vi "Pre Launch Init.vi"(11 "Image Acquisition in":refnum<class "Image Acquisition.lvclass">) -> (0 "error out":errorcluster, 3 "Image Acquisition out":refnum<class "Image Acquisition.lvclass">)   [LabVIEW 2019, in "Image Acquisition.lvlib" / "Image Acquisition.lvclass"]
doc: "(<B>Filename</B>: Actor Framework.lvlib:Actor.lvclass:Pre Launch Init.vi)\n\nDefines behavior that occurs after the Launch Nested Actor method is invoked but before the actor's Actor Core method begins running.\n\nBy default, this method does nothing. A descendant class may override it to define behavior."
uses:
  Image Acquisition.lvclass
  <vilib>/vision/Image Controls.llb/IMAQ Image.ctl
  TypeDefs/Acquired Image Info.ctl
  <vilib>/userdefined/High Color/IMAQdx.ctl
  <vilib>/vision/driver/IMAQdx.llb/IMAQdx Acquisition Mode.ctl
  <vilib>/vision/driver/IMAQdx.llb/IMAQdx Buffer Number Mode.ctl
  TypeDefs/Image Acquisition Parameters.ctl
  TypeDefs/Initialize Data IA.ctl
  <vilib>/ActorFramework/Actor/Actor.lvclass
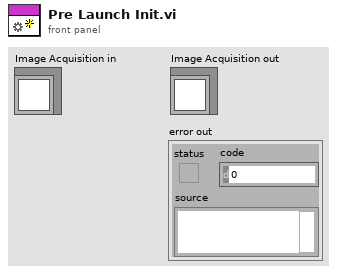
[diagram p1: front panel]
types:
  T1 = typedef "Image Acquisition.lvlib/Image Acquisition.lvclass/Initialize Data IA.ctl" = cluster{"Core":cluster{"Current VI Reference":refnum<vi>, "Close Panel on Exit?":bool}, "IA JSON File Path":path, "Buffer Number":u64, "Missed Frame Count":i32, "Timeout":i32, "Image_Counter_CA":u64, "Imaqdx Session In":T2, "filenames":string[], "File path to read images":path, "Sequence":string, "IMAQ ring Buffer":T3[], "Buffer count":i32, "AOI":i32[], "Offline Images Ring Buffer":T3[], "ReceiverSequence":cluster{"ReceiverID":i32, "Index":i32}[], "Number Of Buffers":i32, "IMAQ Offline Image Buffer":T3[], "IMAQ Run image Buffer ":T3[], "Camera parameters":T4, "CurrentPartParameters":cluster{"Name":string, "ReceiverSequence":cluster{"ReceiverID":dbl, "Index":dbl}[], "AOI":i32[], "filePath":string}, "Exposure Time":u32, "File path @ Run":path, "State Ack":cluster{"State":string, "Status":string}}
  T2 = typedef "IMAQdx.ctl" = refnum<k21>
  T3 = typedef "IMAQ Image.ctl" = refnum<image>
  T4 = typedef "Image Acquisition.lvlib/Image Acquisition.lvclass/Image Acquisition Parameters.ctl" = cluster{"Camera parameters":cluster{"Id":i32, "Type":string, "Model":string, "InterfaceType":string, "SerialNumber":string, "Timeout":i32, "NumberOfBuffers":i32, "AcquisitionTimeout":i32, "ImageName":string, "ColorCameraParam":cluster{"PixelFormat":string, "GammaEnable":bool, "GammaSelector":string, "BalanceRationSelector":string[], "BalanceRationRaw":i32[], "BalanceWhiteAuto":string, "LightSourceSelector":string}, "sessionID":T2, "Continuous?":T5, "Image Type":T6, "Buffer Number Mode (Next)":T7, "PartsList":cluster{"Name":string, "ReceiverSequence":cluster{"ReceiverID":dbl, "Index":dbl}[], "AOI":i32[], "filePath":string}[], "AOI ":i32[], "Default file path":path, "Offline":bool, "GeneralCameraConfig":cluster{"ActiveAttribute":string, "Value":string}[], "DefaultReceiverSequence":cluster{"ReceiverID":dbl, "Index":dbl}[], "Front Panel Open?":bool}, "PartName":string[]}
  T5 = typedef "NI_Vision_Acquisition_Software.lvlib/IMAQdx Acquisition Mode.ctl" = enum32{"One Shot", "Continuous"}
  T6 = typedef "Image Type" = u32
  T7 = typedef "NI_Vision_Acquisition_Software.lvlib/IMAQdx Buffer Number Mode.ctl" = enum32{"Next", "Last", "Buffer Number", "Every", "Last New"}
  T8 = cluster{"Image Acquisition ID":i32, "IA JSON File Path":path}
  T9 = typedef "Image Acquisition.lvlib/Image Acquisition.lvclass/Acquired Image Info.ctl" = cluster{"type":string, "Image Out":T3, "Buffer Number":u64, "Count":u64, "Buffer Count":u64}
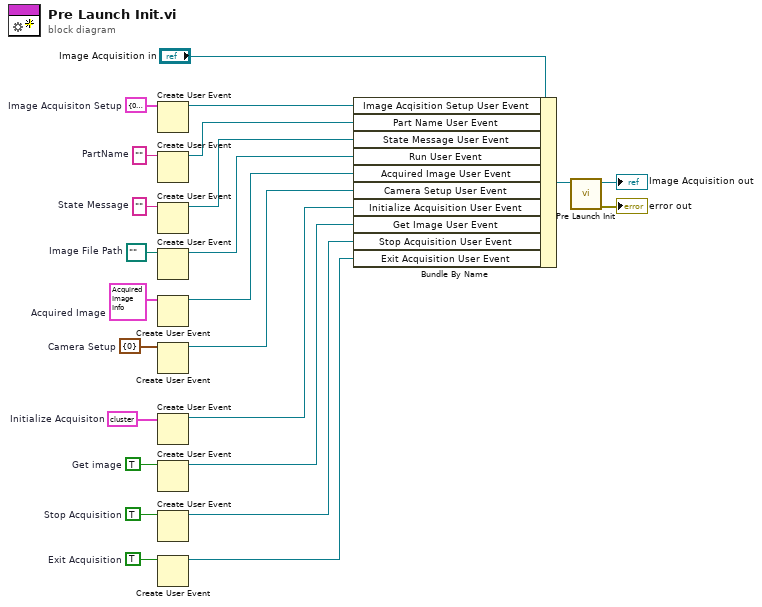
[diagram p0: block diagram]
diagram:
  w2 = cluster{"Initialization Data IA":T1} {"Initialization Data IA"={"Core"={"Current VI Reference"=refnum, "Close Panel on Exit?"=FALSE}, "IA JSON File Path"=path "", "Buffer Number"=0, "Missed Frame Count"=0, "Timeout"=-1, "Image_Counter_CA"=0, "Imaqdx Session In"="", "filenames"=[], "File path to read images"=path "", "Sequence"="", "IMAQ ring Buffer"=[], "Buffer count"=0, "AOI"=[], "Offline Images Ring Buffer"=[], "ReceiverSequence"=[], "Number Of Buffers"=0, "IMAQ Offline Image Buffer"=[], "IMAQ Run image Buffer "=[], "Camera parameters"={"Camera parameters"={"Id"=0, "Type"="", "Model"="", "InterfaceType"="", "SerialNumber"="", "Timeout"=0, "NumberOfBuffers"=0, "AcquisitionTimeout"=0, "ImageName"="", "ColorCameraParam"={"PixelFormat"="", "GammaEnable"=FALSE, "GammaSelector"="", "BalanceRationSelector"=[], "BalanceRationRaw"=[], "BalanceWhiteAuto"="", "LightSourceSelector"=""}, "sessionID"="", "Continuous?"=enum."One Shot", "Image Type"=0, "Buffer Number Mode (Next)"=enum."Next", "PartsList"=[{"Name"="", "ReceiverSequence"=[], "AOI"=[], "filePath"=""}], "AOI "=[], "Default file path"=path "", "Offline"=FALSE, "GeneralCameraConfig"=[], "DefaultReceiverSequence"=[], "Front Panel Open?"=FALSE}, "PartName"=[]}, "CurrentPartParameters"={"Name"="", "ReceiverSequence"=[], "AOI"=[], "filePath"=""}, "Exposure Time"=0, "File path @ Run"=path "", "State Ack"={"State"="", "Status"=""}}}  # Initialize Acquisiton
  w6 = TRUE  # Exit Acquisition
  w7 = TRUE  # Stop Acquisition
  w8 = TRUE  # Get image
  w10 = cluster{"Exposure Time":i32} {"Exposure Time"=0}  # Camera Setup
  w18 = T8 {"Image Acquisition ID"=0, "IA JSON File Path"=path ""}  # Image Acquisiton Setup
  w19 = T9 {"type"="", "Image Out"=refnum, "Buffer Number"=0, "Count"=0, "Buffer Count"=0}  # Acquired Image
  w20 = path ""  # Image File Path
  w21 = ""  # State Message
  w22 = ""  # PartName
  n1 = Create User Event(user event datatype=w18) -> (user event=w17:refnum<user-event>)  [unwired: 1 in, 1 out]
  n2 = Create User Event(user event datatype=w22) -> (user event=w16:refnum<user-event>)  [unwired: 1 in, 1 out]
  n3 = Create User Event(user event datatype=w21) -> (user event=w15:refnum<user-event>)  [unwired: 1 in, 1 out]
  n4 = Create User Event(user event datatype=w20) -> (user event=w14:refnum<user-event>)  [unwired: 1 in, 1 out]
  n5 = Create User Event(user event datatype=w19) -> (user event=w13:refnum<user-event>)  [unwired: 1 in, 1 out]
  n6 = Create User Event(user event datatype=w10) -> (user event=w9:refnum<user-event>)  [unwired: 1 in, 1 out]
  n7 = Create User Event(user event datatype=w2) -> (user event=w1:refnum<user-event>)  [unwired: 1 in, 1 out]
  n8 = Create User Event(user event datatype=w8) -> (user event=w5:refnum<user-event>)  [unwired: 1 in, 1 out]
  n9 = Create User Event(user event datatype=w7) -> (user event=w4:refnum<user-event>)  [unwired: 1 in, 1 out]
  n10 = Create User Event(user event datatype=w6) -> (user event=w3:refnum<user-event>)  [unwired: 1 in, 1 out]
  n11 = Bundle By Name(cluster="Image Acquisition in", "Image Acqisition Setup User Event"=w17, "Part Name User Event"=w16, "State Message User Event"=w15, "Run User Event"=w14, "Acquired Image User Event"=w13, "Camera Setup User Event"=w9, "Initialize Acquisition User Event"=w1, "Get Image User Event"=w5, "Stop Acquisition User Event"=w4, "Exit Acquisition User Event"=w3) -> (w11:refnum<class "Image Acquisition.lvclass">)
  n12 = call-parent "Pre Launch Init.vi"("Actor in"=w11) -> ("error out"=→"error out":errorcluster, "Actor out"=→"Image Acquisition out":refnum<class "Image Acquisition.lvclass">)  [unwired: 9 in]
